vi "Get Instances.vi"(6 "Base Class (LabVIEW Object)":refnum<class>, 8 "error in (no error)":errorcluster, 11 "Lookup Service in":refnum<data-value>) -> (0 "error out":errorcluster, 3 "Lookup Service out":refnum<data-value>, 5 "instances":refnum<data-value>[](array[refnum]))   [LabVIEW 2014, in "LVCOOOP.lvlib" / "Lookup API.lvlib" / "Lookup Service.lvclass"]
doc: "Get all registered instances of the specified base class."
uses:
  Lookup Service.lvclass
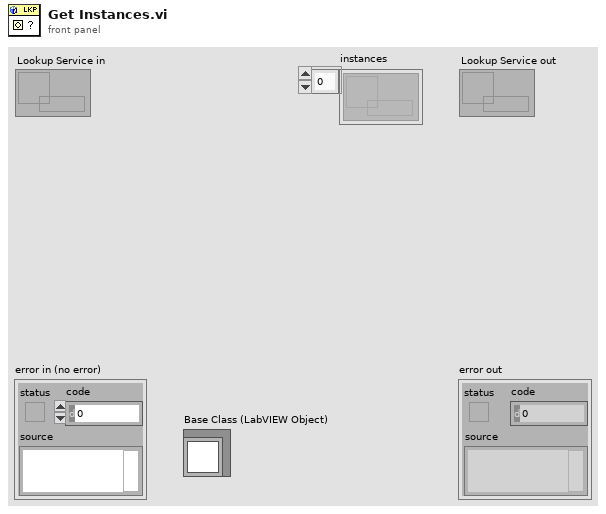
[diagram p1: front panel]
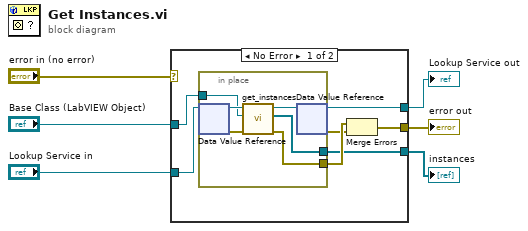
[diagram p0: block diagram]
diagram:
  n1 = case shown="No Error" "error in (no error)" {
    selector: "error in (no error)" -> [_ w20]
    tunnel: "Base Class (LabVIEW Object)" -> [w13 _]
    tunnel: "Lookup Service in" -> [w10 w21]
    tunnel: [w9 w21] -> w4
    tunnel: [w8 w20] -> w3
    tunnel: [w7 _] -> w1
    frame No Error {
      n2 = in-place {
        in-place-border: w13 -> [w16]
        in-place-border: [w19] -> w12
        in-place-border: [w14] -> w7
        n3 = in-place-dvr #1(w10) -> (w18:refnum<class "Lookup Service.lvclass">, w15:errorcluster)
        n4 = call-dynamic "get_instances.vi"("error in (no error)"=w15, "Base Class (LabVIEW Object)"=w16, "Lookup Service in"=w18) -> ("error out"=w19:errorcluster, "instances"=w14:refnum<data-value>[], "Lookup Service out"=w17:refnum<class "Lookup Service.lvclass">)  [unwired: 6 in]
        n5 = in-place-dvr #1(w17) -> (w9:refnum<data-value>, w11:errorcluster)
      }
      n6 = Merge Errors(w12, w11) -> (w8:errorcluster)
    }
    frame Error {
    }
  }
  "error out" <- w3
  "Lookup Service out" <- w4
  "instances" <- w1
